vi "Set Arm.vi"(9 "Arm Mode":T1, 10 "Manual Up":bool, 11 "Manual Down":bool) -> ()   [LabVIEW 2015]
uses:
  Arm Mode TypeDef.ctl
  Arm Notifier TypeDef.ctl
  Global Variables.vi
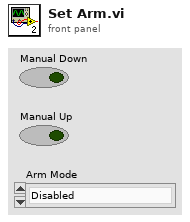
[diagram p1: front panel]
types:
  T1 = typedef "Arm Mode TypeDef.ctl" = enum16{"Disabled", "Locked", "Manual", "Shoot", "Cross Defense", "Low Bar", "Human Player Load"}
  T2 = typedef "Arm Notifier TypeDef.ctl" = cluster{"Arm Mode":T1, "Manual Up":bool, "Manual Down":bool, "Last Update":u32}
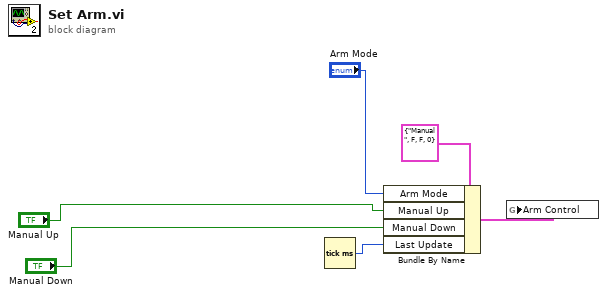
[diagram p0: block diagram]
diagram:
  n1 = Tick Count (ms)() -> (millisecond timer value=w6:u32)
  n2 = Bundle By Name(cluster=T2 {"Arm Mode"=enum."Manual", "Manual Up"=FALSE, "Manual Down"=FALSE, "Last Update"=0} ("Arm Control"), "Arm Mode"="Arm Mode", "Manual Up"="Manual Up", "Manual Down"="Manual Down", "Last Update"=w6) -> (w4:T2)
  n3 = global write "Global Variables.vi" "Arm Control"(w4) -> ()
